vi "FWHM xy graph.vi"(0 "xy graph":cluster{"all rows":dbl[], "all rows":dbl[]}(graph)) -> (1 "FWHM":dbl format="%.2f", 2 "max index(es)":i32, 3 "initial guess":T1={"initial amplitude"=nan, "initial center"=nan, "initial standard deviation"=nan, "offset"=nan})   [LabVIEW 2013]
uses:
  <vilib>/Analysis/baseanly.llb/Mean (DBL).vi
  <vilib>/Analysis/NI_AALBase.lvlib
panel:
  out "peak y/2":dbl
  out "half max rhs pix":dbl
  out "half max lhs pix":dbl
  out "peak y value":dbl
  out "FWHM pix":dbl format="%.2f"
  out "center x value":dbl
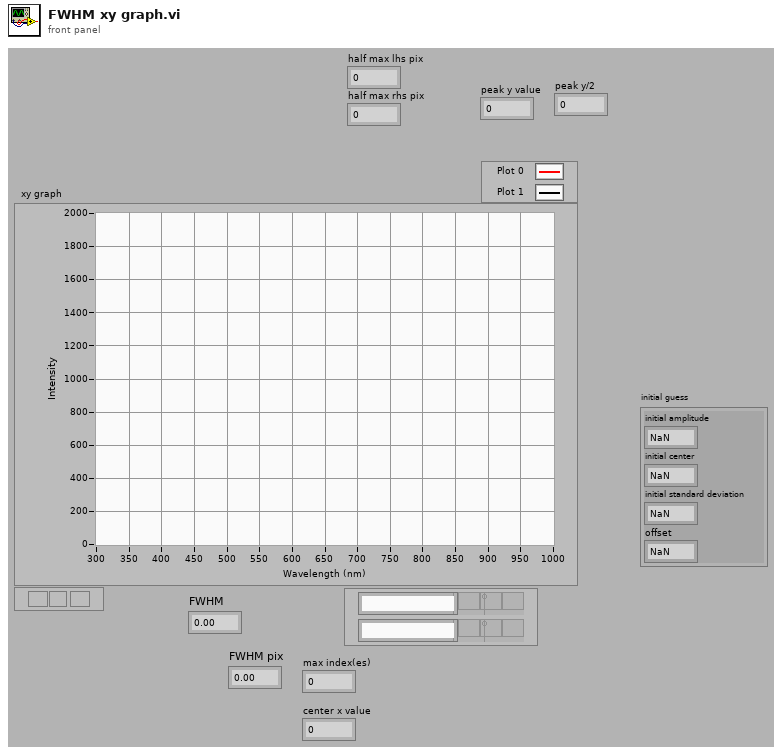
[diagram p1: front panel]
types:
  T1 = cluster{"initial amplitude":dbl, "initial center":dbl, "initial standard deviation":dbl, "offset":dbl}
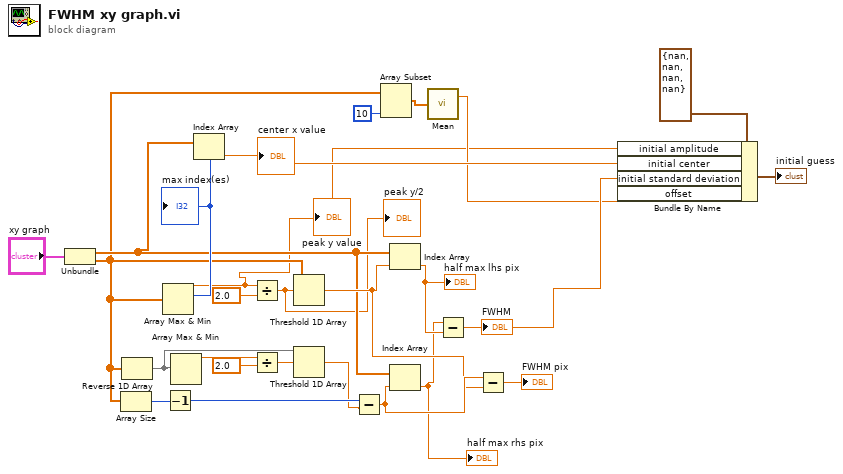
[diagram p0: block diagram]
diagram:
  n1 = Unbundle("xy graph") -> ("all rows"=w8:dbl[], "all rows"=w4:dbl[])
  n2 = Array Size(array=w4) -> (size(s)=w23:i32)
  n3 = Reverse 1D Array(array=w4) -> (reversed array=w22:dbl[])
  n4 = Array Max & Min(array=w4) -> (max value=w2:dbl, max index (indices)=w11:i32)  [unwired: 2 out]
  "max index(es)" <- w11
  "peak y value" <- w2
  n5 = Decrement(x=w23) -> (x-1=w25:i32)
  n6 = Array Max & Min(array=w22) -> (max value=w18:dbl)  [unwired: 3 out]
  n7 = Index Array(array=w8, index=w11) -> (element=w10:dbl)
  "center x value" <- w10
  n8 = Divide(x=w2, y=2.0) -> (x/y=w1:dbl)
  "peak y/2" <- w1
  n9 = Divide(x=w18, y=2.0) -> (x/y=w21:dbl)
  n10 = Threshold 1D Array(2:w1, 3:w4) -> (0:w14:dbl)  [unwired: 1 out]
  n11 = Threshold 1D Array(2:w21, 3:w22) -> (0:w24:dbl)  [unwired: 1 out]
  n12 = Subtract(x=w25, y=w24) -> (x-y=w15:dbl)
  n13 = Array Subset(array=w4, length=10) -> (w6:dbl[])  [unwired: 1 in]
  n14 = Index Array(array=w8, index=w14) -> (element=w17:dbl)
  "half max lhs pix" <- w17
  n15 = Index Array(array=w8, index=w15) -> (element=w3:dbl)
  "half max rhs pix" <- w3
  n16 = call-poly <vilib>:"Mean.vi"("X"=w6) -> ("mean"=w5:dbl)  [unwired: 1 out]
  n17 = Subtract(x=w3, y=w17) -> (x-y=w9:dbl)
  "FWHM" <- w9
  n18 = Subtract(x=w15, y=w14) -> (x-y=→"FWHM pix":dbl)
  n19 = Bundle By Name(cluster=T1 {"initial amplitude"=nan, "initial center"=nan, "initial standard deviation"=nan, "offset"=nan} ("initial guess"), "initial amplitude"=w2, "initial center"=w10, "initial standard deviation"=w9, "offset"=w5) -> (→"initial guess":T1)
